vi "DATA_TO_STR.vi"(8 "ref_File_ErrIn":errorcluster caption="에러 입력", 9 "Index":u32, 10 "DATA":T1(array[cluster]), 11 "ref_File_In":refnum<file>) -> (0 "ref_File_ErrOut":errorcluster caption="에러 출력", 1 "Index_Out":u32, 3 "ref_File_Out":refnum<file>)   [LabVIEW 2019]
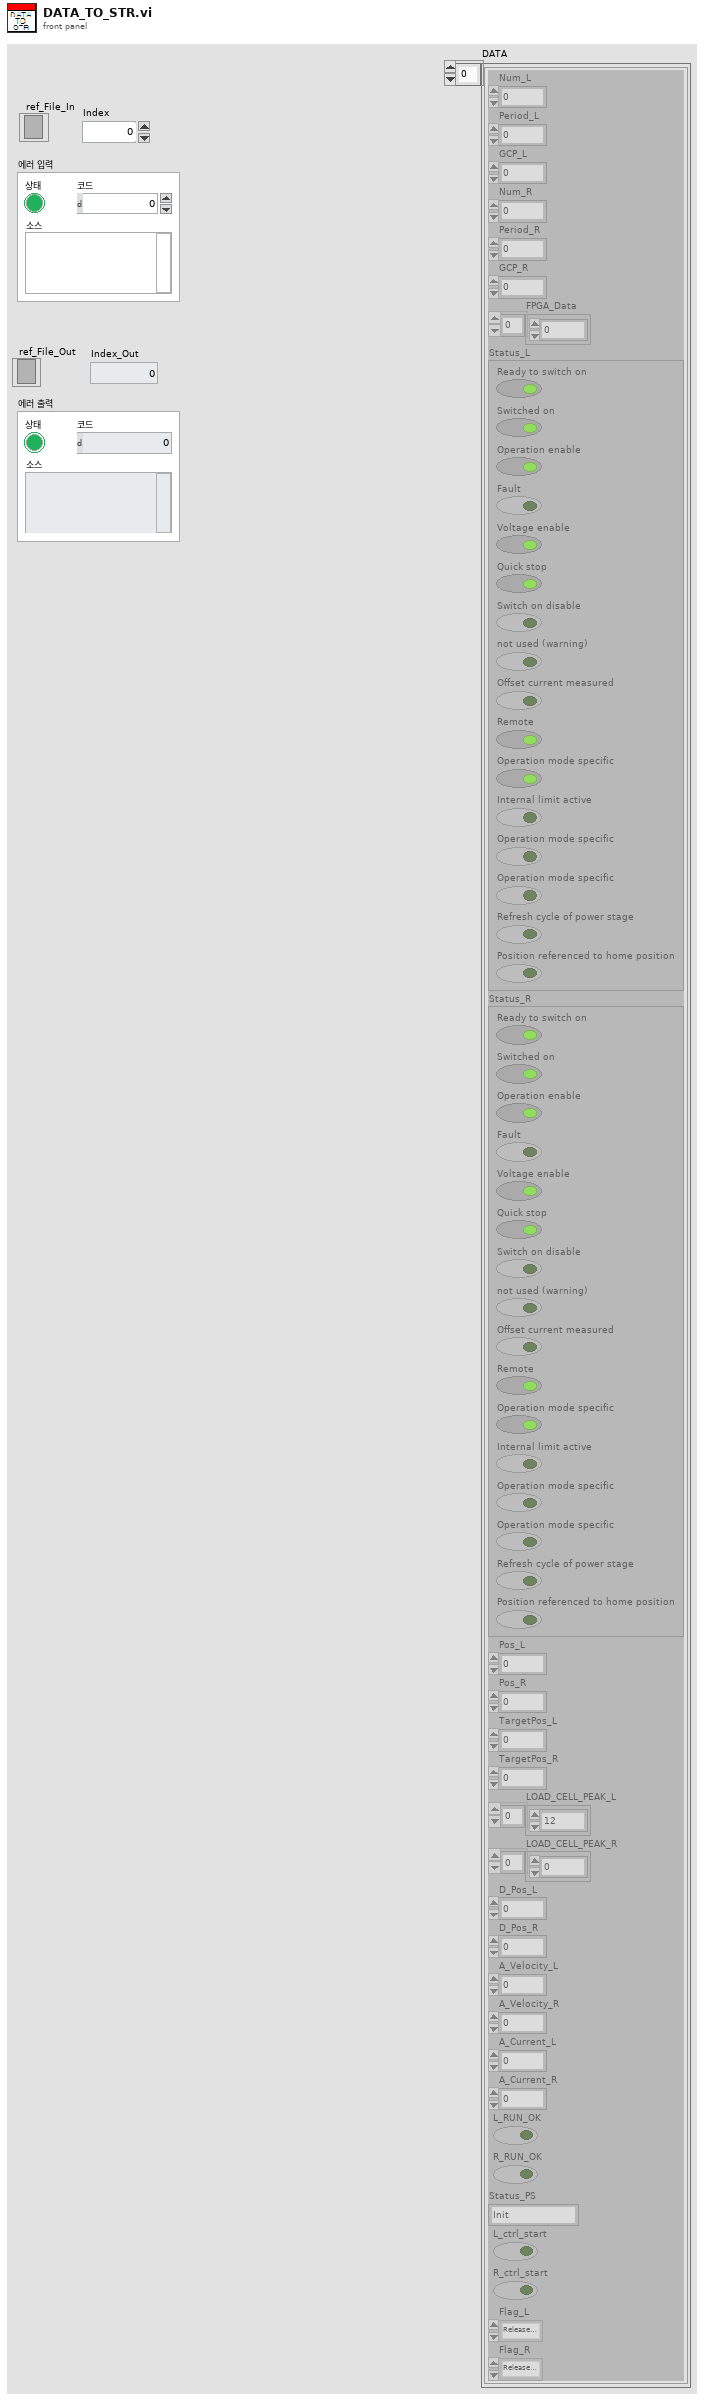
[diagram p1: front panel]
types:
  T1 = cluster{"Num_L":u32, "Period_L":u32, "GCP_L":sgl, "Num_R":u32, "Period_R":u32, "GCP_R":sgl, "FPGA_Data":sgl[], "Status_L":cluster{"Ready to switch on":bool, "Switched on":bool, "Operation enable":bool, "Fault":bool, "Voltage enable":bool, "Quick stop":bool, "Switch on disable":bool, "not used (warning)":bool, "Offset current measured":bool, "Remote":bool, "Operation mode specific":bool, "Internal limit active":bool, "Operation mode specific":bool, "Operation mode specific":bool, "Refresh cycle of power stage":bool, "Position referenced to home position":bool}, "Status_R":cluster{"Ready to switch on":bool, "Switched on":bool, "Operation enable":bool, "Fault":bool, "Voltage enable":bool, "Quick stop":bool, "Switch on disable":bool, "not used (warning)":bool, "Offset current measured":bool, "Remote":bool, "Operation mode specific":bool, "Internal limit active":bool, "Operation mode specific":bool, "Operation mode specific":bool, "Refresh cycle of power stage":bool, "Position referenced to home position":bool}, "Pos_L":i32, "Pos_R":i32, "TargetPos_L":i32, "TargetPos_R":i32, "LOAD_CELL_PEAK_L":sgl[], "LOAD_CELL_PEAK_R":sgl[], "D_Pos_L":i32, "D_Pos_R":i32, "A_Velocity_L":i32, "A_Velocity_R":i32, "A_Current_L":i16, "A_Current_R":i16, "L_RUN_OK":bool, "R_RUN_OK":bool, "Status_PS":string, "L_ctrl_start":bool, "R_ctrl_start":bool, "Flag_L":enum16{"Release_start", "Calculate", "Onset_start", "Peak_start"}, "Flag_R":enum16{"Release_start", "Calculate", "Onset_start", "Peak_start"}}[]
  T2 = enum16{"Release_start", "Calculate", "Onset_start", "Peak_start"}
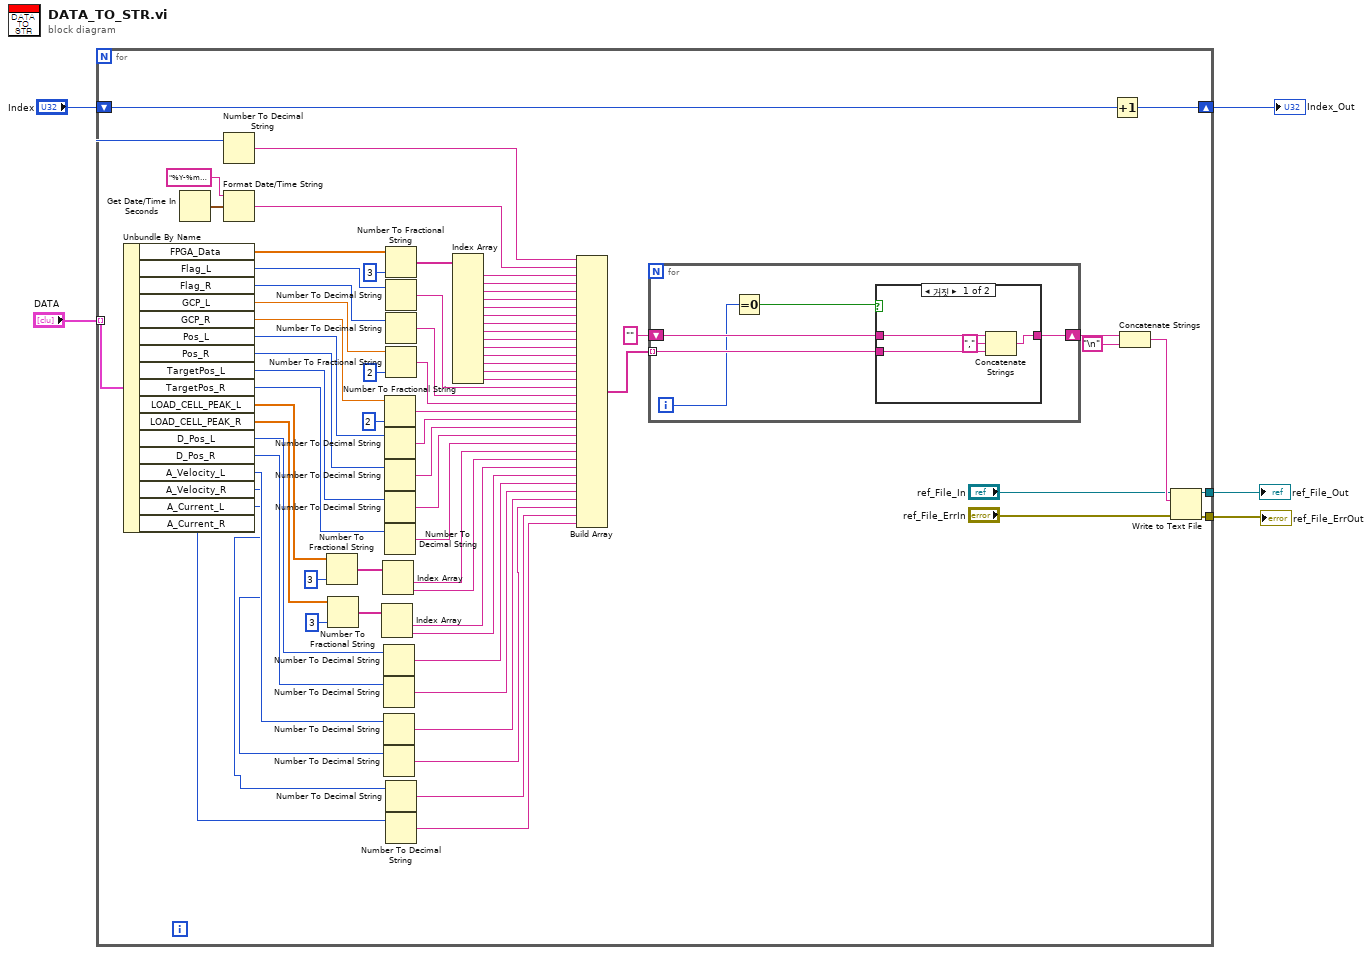
[diagram p0: block diagram]
diagram:
  n1 = for {
    tunnel: [w64] -> w5
    tunnel: [w63] -> w4
    tunnel: "DATA" -> [w59] mode=indexing
    shift-right: [w60] -> w2
    shift-left: "Index" -> [w61]
    n2 = Unbundle By Name(w59) -> ("FPGA_Data"=w76:sgl[], "Flag_L"=w70:T2, "Flag_R"=w69:T2, "GCP_L"=w67:sgl, "GCP_R"=w66:sgl, "Pos_L"=w58:i32, "Pos_R"=w57:i32, "TargetPos_L"=w56:i32, "TargetPos_R"=w55:i32, "LOAD_CELL_PEAK_L"=w26:sgl[], "LOAD_CELL_PEAK_R"=w23:sgl[], "D_Pos_L"=w17:i32, "D_Pos_R"=w16:i32, "A_Velocity_L"=w13:i32, "A_Velocity_R"=w8:i32, "A_Current_L"=w7:i16, "A_Current_R"=w6:i16)
    n3 = Get Date/Time In Seconds() -> (seconds since 1Jan1904=w78:timestamp)
    n4 = Number To Decimal String(number=w61) -> (decimal integer string=w72:string)  [unwired: 1 in]
    n5 = Format Date/Time String(time format string (%c)="%Y-%m-%d_%H%M%S_%3u" ("시간 포맷 문자열 (%c)"), seconds (now)=w78) -> (date/time string=w73:string)  [unwired: 1 in]
    n6 = Number To Fractional String(number=w26, precision (6)=i16 3 ("정밀도(6)")) -> (F-format string=w25:string[])  [unwired: 2 in]
    n7 = Number To Fractional String(number=w23, precision (6)=i16 3 ("정밀도(6)")) -> (F-format string=w22:string[])  [unwired: 2 in]
    n8 = Index Array(array=w22) -> (element #1=w19:string, element #2=w18:string)  [unwired: 2 in]
    n9 = Index Array(array=w25) -> (element #1=w21:string, element #2=w20:string)  [unwired: 2 in]
    n10 = Number To Decimal String(number=w17) -> (decimal integer string=w15:string)  [unwired: 1 in]
    n11 = Number To Decimal String(number=w16) -> (decimal integer string=w14:string)  [unwired: 1 in]
    n12 = Number To Decimal String(number=w13) -> (decimal integer string=w12:string)  [unwired: 1 in]
    n13 = Number To Decimal String(number=w8) -> (decimal integer string=w11:string)  [unwired: 1 in]
    n14 = Number To Fractional String(number=w66, precision (6)=i16 2 ("정밀도(6)")) -> (F-format string=w33:string)  [unwired: 2 in]
    n15 = Number To Decimal String(number=w58) -> (decimal integer string=w32:string)  [unwired: 1 in]
    n16 = Number To Decimal String(number=w57) -> (decimal integer string=w31:string)  [unwired: 1 in]
    n17 = Number To Decimal String(number=w56) -> (decimal integer string=w30:string)  [unwired: 1 in]
    n18 = Number To Decimal String(number=w55) -> (decimal integer string=w29:string)  [unwired: 1 in]
    n19 = Number To Fractional String(number=w76, precision (6)=i16 3 ("정밀도(6)")) -> (F-format string=w75:string[])  [unwired: 2 in]
    n20 = Number To Decimal String(number=w70) -> (decimal integer string=w36:string)  [unwired: 1 in]
    n21 = Number To Decimal String(number=w69) -> (decimal integer string=w35:string)  [unwired: 1 in]
    n22 = Number To Fractional String(number=w67, precision (6)=i16 2 ("정밀도(6)")) -> (F-format string=w34:string)  [unwired: 2 in]
    n23 = Number To Decimal String(number=w7) -> (decimal integer string=w10:string)  [unwired: 1 in]
    n24 = Number To Decimal String(number=w6) -> (decimal integer string=w9:string)  [unwired: 1 in]
    n25 = Index Array(array=w75) -> (element #1=w50:string, element #2=w49:string, element #3=w48:string, element #4=w47:string, element #5=w46:string, element #6=w45:string, element #7=w44:string, element #8=w43:string, element #9=w42:string, element #10=w41:string, element #11=w40:string, element #12=w39:string, element #13=w38:string, element #14=w37:string)  [unwired: 14 in]
    n26 = Build Array(w72, w73, w50, w49, w48, w47, w46, w45, w44, w43, w42, w41, w40, w39, w38, w37, w36, w35, w34, w33, w32, w31, w30, w29, w21, w20, w19, w18, w15, w14, w12, w11, w10, w9) -> (w65:string[])
    n27 = for {
      tunnel: w65 -> [w82] mode=indexing
      shift-right: [w81] -> w54
      shift-left: "" -> [w83]
      i -> [w79]
      n28 = Equal To 0?(x=w79) -> (x = 0?=w80:bool)
      n29 = case shown="거짓" w80 {
        tunnel: w83 -> [w87 _]
        tunnel: w82 -> [w85 w88]
        tunnel: [w84 w88] -> w81
        frame False {
          n30 = Concatenate Strings(w87, "," ("문자열"), w85) -> (w84:string)
        }
        frame True {
        }
      }
    }
    n31 = Increment(x=w61) -> (x+1=w60:u32)
    n32 = Concatenate Strings(w54, "\n") -> (w53:string)
    n33 = Write to Text File ("텍스트 파일에 쓰기")(file (use dialog)="ref_File_In", text=w53, error in="ref_File_ErrIn") -> (refnum out=w64:refnum<file>, error out=w63:errorcluster)  [unwired: 1 in, 1 out]
  }
  "ref_File_Out" <- w5
  "ref_File_ErrOut" <- w4
  "Index_Out" <- w2
